vi "Resistor CalculatorLV2012 NIVerified.vi"() -> ()   [LabVIEW 2012]
doc: "This VI will calculate the value of your resistor based on the colors of the bands on your resistor. Each tab will show the meaning of each band of your resistor. When you are finished, you will find the nominal value of the resistor, the tolerance value on your resistor, the change in resistance caused by temperature and the maximum and minimum values that your resistance can be. \n\n1.) Select your resistor style from the tabs above.\n2.) Select the specific colors that are on your resistor.\n3.) If you are using a 6 Band resistor, enter the operating temperature of the resistor to determine the additional resistance caused by the change in temperature.\n4.) Click \"Calculate\" to determine the resulting resistor values."
panel:
  in  "Stop":bool
  in  "Calculate":bool
  in  "Tab Control":T1(tab)
  in  "1st Digit":u16(ring)=1 items=["Black", "Brown", "Red", "Orange", "Yellow", "Green", "Blue", "Purple", "Grey", "White"]
  in  "2nd Digit":u16(ring)=1 items=["Black", "Brown", "Red", "Orange", "Yellow", "Green", "Blue", "Purple", "Grey", "White"]
  in  "Multiplier":dbl(ring)=10.0 items=["Silver"=0.01, "Gold"=0.1, "Black"=1.0, "Brown"=10.0, "Red"=100.0, "Orange"=1000.0, "Yellow"=10000.0, "Green"=100000.0, "Blue"=1000000.0, "Purple"=10000000.0]
  in  "Tolerance":dbl(ring)=0.01 items=["Silver"=0.1, "Gold"=0.05, "Brown"=0.01, "Red"=0.02, "Green"=0.005, "Blue"=0.0025, "Purple"=0.001]
  out "1":bool
  out "2":bool
  out "Mult":bool
  out "Tol":bool
  out "Mult 2":bool
  out "1 2":bool
  out "2 2":bool
  out "3 2":bool
  out "Tol 2":bool
  in  "1st Digit":u16(ring)=1 items=["Black", "Brown", "Red", "Orange", "Yellow", "Green", "Blue", "Purple", "Grey", "White"]
  in  "2nd Digit":u16(ring)=1 items=["Black", "Brown", "Red", "Orange", "Yellow", "Green", "Blue", "Purple", "Grey", "White"]
  in  "Multiplier":dbl(ring)=10.0 items=["Silver"=0.01, "Gold"=0.1, "Black"=1.0, "Brown"=10.0, "Red"=100.0, "Orange"=1000.0, "Yellow"=10000.0, "Green"=100000.0, "Blue"=1000000.0, "Purple"=10000000.0]
  in  "Tolerance":dbl(ring)=0.01 items=["Silver"=0.1, "Gold"=0.05, "Brown"=0.01, "Red"=0.02, "Green"=0.005, "Blue"=0.0025, "Purple"=0.001]
  in  "3rd Digit":u16(ring)=1 items=["Black", "Brown", "Red", "Orange", "Yellow", "Green", "Blue", "Purple", "Grey", "White"]
  in  "Temperature (C)":dbl=25.0
  out "Temp 3":bool
  out "Mult 3":bool
  out "1 3":bool
  out "23":bool
  out "33":bool
  out "Tol 3":bool
  in  "1st Digit":u16(ring)=1 items=["Black", "Brown", "Red", "Orange", "Yellow", "Green", "Blue", "Purple", "Grey", "White"]
  in  "2nd Digit":u16(ring)=1 items=["Black", "Brown", "Red", "Orange", "Yellow", "Green", "Blue", "Purple", "Grey", "White"]
  in  "Multiplier":dbl(ring)=10.0 items=["Silver"=0.01, "Gold"=0.1, "Black"=1.0, "Brown"=10.0, "Red"=100.0, "Orange"=1000.0, "Yellow"=10000.0, "Green"=100000.0, "Blue"=1000000.0, "Purple"=10000000.0]
  in  "Tolerance":dbl(ring)=0.01 items=["Silver"=0.1, "Gold"=0.05, "Brown"=0.01, "Red"=0.02, "Green"=0.005, "Blue"=0.0025, "Purple"=0.001]
  in  "3rd Digit":u16(ring)=1 items=["Black", "Brown", "Red", "Orange", "Yellow", "Green", "Blue", "Purple", "Grey", "White"]
  in  "Temp Coefficient":i32(ring)=100 items=["Brown"=100, "Red"=50, "Orange"=15, "Yellow"=25, "Blue"=10, "Purple"=5]
  out "Resistor Value":dbl=110.0 format="%#_6p"
  out "Tolerance Value":dbl=1.1 format="%#_6p"
  out "Lowest Actual Value":dbl=108.9 format="%#_6p"
  out "Highest Actual Value":dbl=111.1 format="%#_6p"
  out "Temp Adjustment":dbl format="%#_6p"
  # "Overview: To demonstrate how to set up a simple analog window\nRequirement: LabVIEW Full Development System\nSteps:\n1. Choose how many bands do you want to calculate\n2. Set the color.\n3. Run the VI"
  # "This VI will calculate the value of your resistor based on the colors of the bands on your resistor. Each tab will show the meaning of each band of your resistor. When you are finished, you will find the nominal value of the resistor, the tolerance value on your resistor, the change in resistance caused by temperature and the maximum and minimum values that your resistance can be. \n\n1.) Select your resistor style from the tabs above.\n2.) Select the specific colors that are on your resistor.\n3.) If you are using a 6 Band resistor, enter the operating temperature of the resistor to determine the additional resistance caused by the change in temperature.\n4.) Click \"Calculate\" to determine the resulting resistor values."
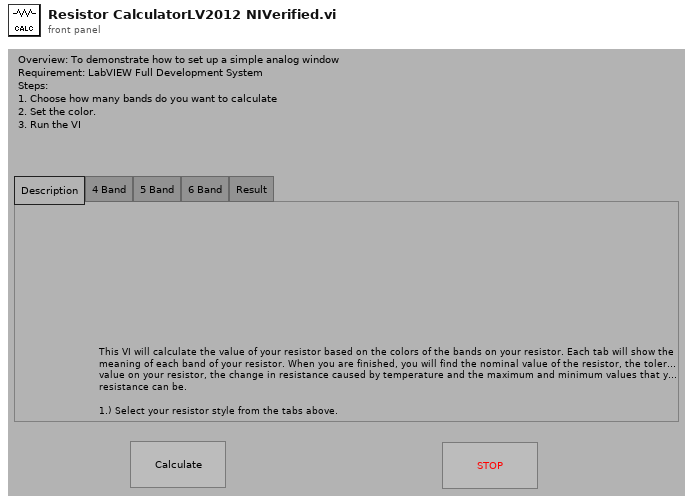
[diagram p1: front panel]
types:
  T1 = enum32{"Description", "4 Band", "5 Band", "6 Band", "Result"}
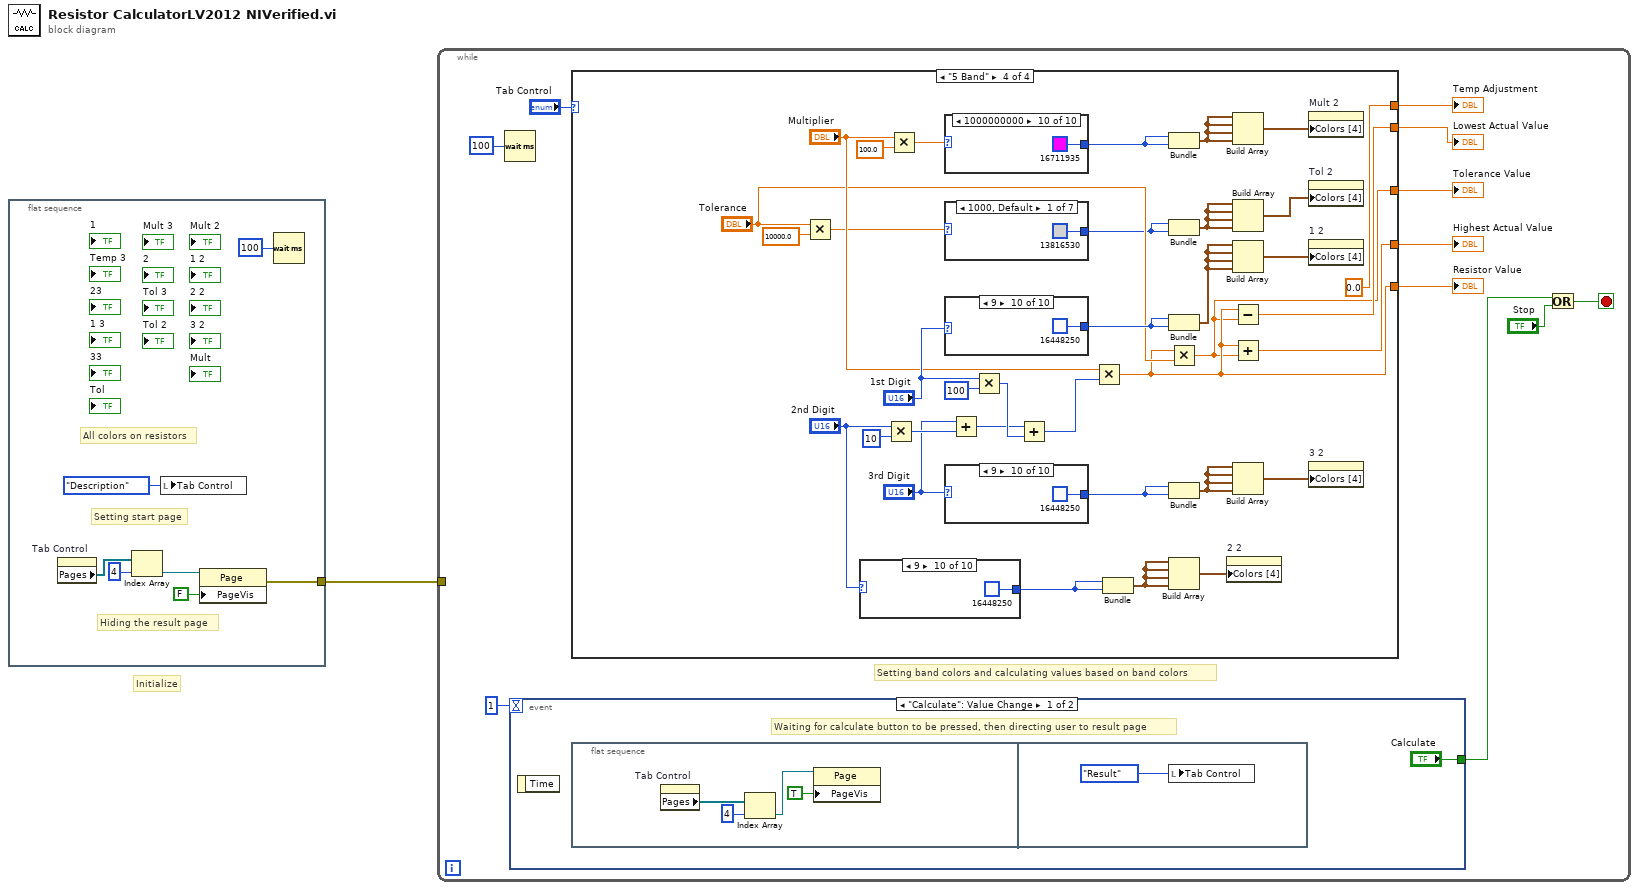
[diagram p0: block diagram]
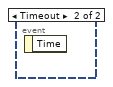
[diagram p2: hidden frame]
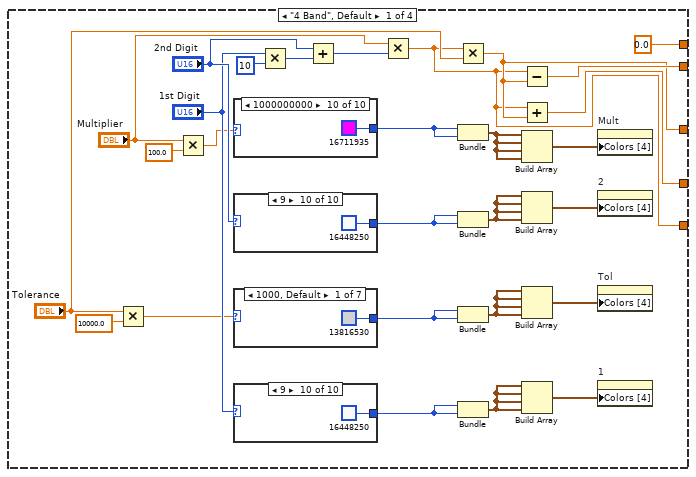
[diagram p3: hidden frame]
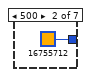
[diagram p4: hidden frame]
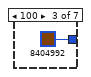
[diagram p5: hidden frame]
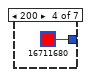
[diagram p6: hidden frame]
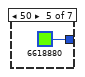
[diagram p7: hidden frame]
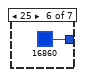
[diagram p8: hidden frame]
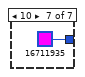
[diagram p9: hidden frame]
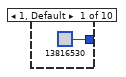
[diagram p10: hidden frame]
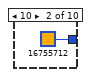
[diagram p11: hidden frame]
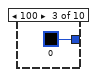
[diagram p12: hidden frame]
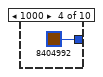
[diagram p13: hidden frame]
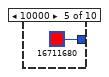
[diagram p14: hidden frame]
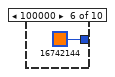
[diagram p15: hidden frame]
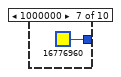
[diagram p16: hidden frame]
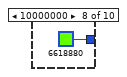
[diagram p17: hidden frame]
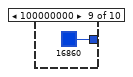
[diagram p18: hidden frame]
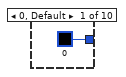
[diagram p19: hidden frame]
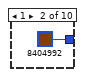
[diagram p20: hidden frame]
diagram:
  # "Initialize"
  n1 = flat-sequence {
    tunnel: [w2] -> w1
    frame #0 {
      # "Hiding the result page"
      # "Setting start page"
      # "All colors on resistors"
      n2 = property on="Tab Control" class="TabCtl (strict)"() -> ("Pages"=w3:refnum<vi>[])  [unwired: 2 in, 2 out]
      n3 = Index Array(array=w3, index=4) -> (element=w4:refnum<vi>)
      n4 = local write "Tab Control"(T1."Description" ("Tab Control")) -> ()
      n5 = property class="Page"(reference=w4, "PageVis"=FALSE ("Page Visible")) -> (error out=w2:errorcluster)  [unwired: 1 in, 1 out]
      n6 = Wait (ms)(milliseconds to wait=u32 100) -> ()  [unwired: 1 out]
    }
  }
  n7 = while {
    tunnel: w1 -> [_]
    stop <- w10 stop-if-true
    # "Setting band colors and calculating values based on band colors"
    n8 = Wait (ms)(milliseconds to wait=u32 100) -> ()  [unwired: 1 out]
    n9 = event shown="[0] \"Calculate\": Value Change" {
      selector: _ -> [_ _]
      dyn-events: _ -> [_ _]
      timeout: 1 -> [_ _]
      tunnel: ["Calculate" _] -> w18
      event "Calculate": Value Change {
        # "Waiting for calculate button to be pressed, then directing user to result page"
        n10 = event-data() -> ()  [unwired: 1 in, 1 out]
        n11 = flat-sequence {
          frame #0 {
            n12 = property on="Tab Control" class="TabCtl (strict)"() -> ("Pages"=w24:refnum<vi>[])  [unwired: 2 in, 2 out]
            n13 = Index Array(array=w24, index=4) -> (element=w23:refnum<vi>)
            n14 = property class="Page"(reference=w23, "PageVis"=TRUE ("Page Visible")) -> ()  [unwired: 1 in, 2 out]
          }
          frame #1 {
            n15 = local write "Tab Control"(T1."Result" ("Tab Control")) -> ()
          }
        }
      }
      event Timeout {
        n16 = event-data() -> ()  [unwired: 1 in, 1 out]
      }
    }
    n17 = case shown="\"5 Band\"" "Tab Control" {
      tunnel: [w30 w107 w186 w200] -> w17
      tunnel: [w29 w106 w186 w199] -> w16
      tunnel: [w28 w105 w186 w198] -> w15
      tunnel: [w27 w98 w186 w201] -> w14
      tunnel: [0.0 w100 w186 0.0] -> w13
      frame "4 Band", Default {
        n18 = Multiply(x="Tolerance", y=10000.0) -> (x*y=w36:dbl)
        n19 = Multiply(x="Multiplier", y=100.0) -> (x*y=w37:dbl)
        n20 = case shown="1000000000" w37 {
          tunnel: [u32 13816530 ("Color Box") u32 16755712 ("Color Box") u32 0 ("Color Box") u32 8404992 ("Color Box") u32 16711680 ("Color Box") u32 16742144 ("Color Box") u32 16776960 ("Color Box") u32 6618880 ("Color Box") u32 16860 ("Color Box") u32 16711935 ("Color Box")] -> w40
          frame 1, Default {
          }
          frame 10 {
          }
          frame 100 {
          }
          frame 1000 {
          }
          frame 10000 {
          }
          frame 100000 {
          }
          frame 1000000 {
          }
          frame 10000000 {
          }
          frame 100000000 {
          }
          frame 1000000000 {
          }
        }
        n21 = case shown="9" "2nd Digit" {
          tunnel: [u32 0 ("Color Box") u32 8404992 ("Color Box") u32 16711680 ("Color Box") u32 16742144 ("Color Box") u32 16776960 ("Color Box") u32 6618880 ("Color Box") u32 16860 ("Color Box") u32 16711935 ("Color Box") u32 12369084 ("Color Box") u32 16448250 ("Color Box")] -> w46
          frame 0, Default {
          }
          frame 1 {
          }
          frame 2 {
          }
          frame 3 {
          }
          frame 4 {
          }
          frame 5 {
          }
          frame 6 {
          }
          frame 7 {
          }
          frame 8 {
          }
          frame 9 {
          }
        }
        n22 = case shown="1000, Default" w36 {
          tunnel: [u32 13816530 ("Color Box") u32 16755712 ("Color Box") u32 8404992 ("Color Box") u32 16711680 ("Color Box") u32 6618880 ("Color Box") u32 16860 ("Color Box") u32 16711935 ("Color Box")] -> w32
          frame 1000, Default {
          }
          frame 500 {
          }
          frame 100 {
          }
          frame 200 {
          }
          frame 50 {
          }
          frame 25 {
          }
          frame 10 {
          }
        }
        n23 = case shown="9" "1st Digit" {
          tunnel: [u32 0 ("Color Box") u32 8404992 ("Color Box") u32 16711680 ("Color Box") u32 16742144 ("Color Box") u32 16776960 ("Color Box") u32 6618880 ("Color Box") u32 16860 ("Color Box") u32 16711935 ("Color Box") u32 12369084 ("Color Box") u32 16448250 ("Color Box")] -> w50
          frame 0, Default {
          }
          frame 1 {
          }
          frame 2 {
          }
          frame 3 {
          }
          frame 4 {
          }
          frame 5 {
          }
          frame 6 {
          }
          frame 7 {
          }
          frame 8 {
          }
          frame 9 {
          }
        }
        n24 = Multiply(x="1st Digit", y=10) -> (x*y=w52:i32)
        n25 = Add(x="2nd Digit", y=w52) -> (x+y=w51:i32)
        n26 = Multiply(x="Multiplier", y=w51) -> (x*y=w27:dbl)
        n27 = Multiply(x=w27, y="Tolerance") -> (x*y=w28:dbl)
        n28 = Bundle("Color Box"=w40, "Color Box"=w40) -> (w39:cluster{"Color Box":u32, "Color Box":u32})  [unwired: 1 in]
        n29 = Bundle("Color Box"=w46, "Color Box"=w46) -> (w47:cluster{"Color Box":u32, "Color Box":u32})  [unwired: 1 in]
        n30 = Bundle("Color Box"=w32, "Color Box"=w32) -> (w33:cluster{"Color Box":u32, "Color Box":u32})  [unwired: 1 in]
        n31 = Bundle("Color Box"=w50, "Color Box"=w50) -> (w49:cluster{"Color Box":u32, "Color Box":u32})  [unwired: 1 in]
        n32 = Subtract(x=w27, y=w28) -> (x-y=w29:dbl)
        n33 = Add(x=w27, y=w28) -> (x+y=w30:dbl)
        n34 = Build Array(w39, w39, w39, w39) -> (w38:cluster{"Color Box":u32, "Color Box":u32}[])
        n35 = Build Array(w47, w47, w47, w47) -> (w45:cluster{"Color Box":u32, "Color Box":u32}[])
        n36 = Build Array(w33, w33, w33, w33) -> (w31:cluster{"Color Box":u32, "Color Box":u32}[])
        n37 = Build Array(w49, w49, w49, w49) -> (w48:cluster{"Color Box":u32, "Color Box":u32}[])
        n38 = property on="Mult" class="Bool (strict)"("Colors [4]"=w38) -> ()  [unwired: 2 in, 2 out]
        n39 = property on="2" class="Bool (strict)"("Colors [4]"=w45) -> ()  [unwired: 2 in, 2 out]
        n40 = property on="Tol" class="Bool (strict)"("Colors [4]"=w31) -> ()  [unwired: 2 in, 2 out]
        n41 = property on="1" class="Bool (strict)"("Colors [4]"=w48) -> ()  [unwired: 2 in, 2 out]
      }
      frame "6 Band" {
        n42 = case shown="9" "2nd Digit" {
          tunnel: [u32 0 ("Color Box") u32 8404992 ("Color Box") u32 16711680 ("Color Box") u32 16742144 ("Color Box") u32 16776960 ("Color Box") u32 6618880 ("Color Box") u32 16860 ("Color Box") u32 16711935 ("Color Box") u32 12369084 ("Color Box") u32 16448250 ("Color Box")] -> w127
          frame 0, Default {
          }
          frame 1 {
          }
          frame 2 {
          }
          frame 3 {
          }
          frame 4 {
          }
          frame 5 {
          }
          frame 6 {
          }
          frame 7 {
          }
          frame 8 {
          }
          frame 9 {
          }
        }
        n43 = Multiply(x="2nd Digit", y=10) -> (x*y=w93:i32)
        n44 = case shown="9" "3rd Digit" {
          tunnel: [u32 0 ("Color Box") u32 8404992 ("Color Box") u32 16711680 ("Color Box") u32 16742144 ("Color Box") u32 16776960 ("Color Box") u32 6618880 ("Color Box") u32 16860 ("Color Box") u32 16711935 ("Color Box") u32 12369084 ("Color Box") u32 16448250 ("Color Box")] -> w112
          frame 0, Default {
          }
          frame 1 {
          }
          frame 2 {
          }
          frame 3 {
          }
          frame 4 {
          }
          frame 5 {
          }
          frame 6 {
          }
          frame 7 {
          }
          frame 8 {
          }
          frame 9 {
          }
        }
        n45 = case shown="9" "1st Digit" {
          tunnel: [u32 0 ("Color Box") u32 8404992 ("Color Box") u32 16711680 ("Color Box") u32 16742144 ("Color Box") u32 16776960 ("Color Box") u32 6618880 ("Color Box") u32 16860 ("Color Box") u32 16711935 ("Color Box") u32 12369084 ("Color Box") u32 16448250 ("Color Box")] -> w131
          frame 0, Default {
          }
          frame 1 {
          }
          frame 2 {
          }
          frame 3 {
          }
          frame 4 {
          }
          frame 5 {
          }
          frame 6 {
          }
          frame 7 {
          }
          frame 8 {
          }
          frame 9 {
          }
        }
        n46 = Multiply(x="1st Digit", y=100) -> (x*y=w92:i32)
        n47 = Compound Arithmetic op=ADD("3rd Digit", w93, w92) -> (w91:i32)
        n48 = Multiply(x="Tolerance", y=10000.0) -> (x*y=w119:dbl)
        n49 = case shown="100, Default" "Temp Coefficient" {
          tunnel: [u32 8404992 ("Color Box") u32 16711680 ("Color Box") u32 16742144 ("Color Box") u32 16776960 ("Color Box") u32 16860 ("Color Box") u32 16711935 ("Color Box")] -> w103
          frame 100, Default {
          }
          frame 50 {
          }
          frame 15 {
          }
          frame 25 {
          }
          frame 10 {
          }
          frame 5 {
          }
        }
        n50 = Multiply(x="Multiplier", y=w91) -> (x*y=w98:dbl)
        n51 = Bundle("Color Box"=w127, "Color Box"=w127) -> (w128:cluster{"Color Box":u32, "Color Box":u32})  [unwired: 1 in]
        n52 = Multiply(x="Multiplier", y=100.0) -> (x*y=w120:dbl)
        n53 = Compound Arithmetic op=MULTIPLY("Temp Coefficient", "Temperature (C)", w98) -> (w95:dbl)
        n54 = case shown="1000000000" w120 {
          tunnel: [u32 13816530 ("Color Box") u32 16755712 ("Color Box") u32 0 ("Color Box") u32 8404992 ("Color Box") u32 16711680 ("Color Box") u32 16742144 ("Color Box") u32 16776960 ("Color Box") u32 6618880 ("Color Box") u32 16860 ("Color Box") u32 16711935 ("Color Box")] -> w122
          frame 1, Default {
          }
          frame 10 {
          }
          frame 100 {
          }
          frame 1000 {
          }
          frame 10000 {
          }
          frame 100000 {
          }
          frame 1000000 {
          }
          frame 10000000 {
          }
          frame 100000000 {
          }
          frame 1000000000 {
          }
        }
        n55 = case shown="1000, Default" w119 {
          tunnel: [u32 13816530 ("Color Box") u32 16755712 ("Color Box") u32 8404992 ("Color Box") u32 16711680 ("Color Box") u32 6618880 ("Color Box") u32 16860 ("Color Box") u32 16711935 ("Color Box")] -> w115
          frame 1000, Default {
          }
          frame 500 {
          }
          frame 100 {
          }
          frame 200 {
          }
          frame 50 {
          }
          frame 25 {
          }
          frame 10 {
          }
        }
        n56 = Build Array(w128, w128, w128, w128) -> (w126:cluster{"Color Box":u32, "Color Box":u32}[])
        n57 = Bundle("Color Box"=w112, "Color Box"=w112) -> (w113:cluster{"Color Box":u32, "Color Box":u32})  [unwired: 1 in]
        n58 = Bundle("Color Box"=w131, "Color Box"=w131) -> (w130:cluster{"Color Box":u32, "Color Box":u32})  [unwired: 1 in]
        n59 = property on="23" class="Bool (strict)"("Colors [4]"=w126) -> ()  [unwired: 2 in, 2 out]
        n60 = Build Array(w113, w113, w113, w113) -> (w114:cluster{"Color Box":u32, "Color Box":u32}[])
        n61 = Build Array(w130, w130, w130, w130) -> (w129:cluster{"Color Box":u32, "Color Box":u32}[])
        n62 = property on="33" class="Bool (strict)"("Colors [4]"=w114) -> ()  [unwired: 2 in, 2 out]
        n63 = property on="1 3" class="Bool (strict)"("Colors [4]"=w129) -> ()  [unwired: 2 in, 2 out]
        n64 = Divide(x=w95, y=1000000.0) -> (x/y=w100:dbl)
        n65 = Bundle("Color Box"=w103, "Color Box"=w103) -> (w104:cluster{"Color Box":u32, "Color Box":u32})  [unwired: 1 in]
        n66 = Add(x=w100, y=w98) -> (x+y=w99:dbl)
        n67 = Build Array(w104, w104, w104, w104) -> (w102:cluster{"Color Box":u32, "Color Box":u32}[])
        n68 = Bundle("Color Box"=w122, "Color Box"=w122) -> (w121:cluster{"Color Box":u32, "Color Box":u32})  [unwired: 1 in]
        n69 = Multiply(x=w98, y="Tolerance") -> (x*y=w105:dbl)
        n70 = Bundle("Color Box"=w115, "Color Box"=w115) -> (w116:cluster{"Color Box":u32, "Color Box":u32})  [unwired: 1 in]
        n71 = property on="Temp 3" class="Bool (strict)"("Colors [4]"=w102) -> ()  [unwired: 2 in, 2 out]
        n72 = Build Array(w121, w121, w121, w121) -> (w109:cluster{"Color Box":u32, "Color Box":u32}[])
        n73 = Subtract(x=w99, y=w105) -> (x-y=w106:dbl)
        n74 = Add(x=w99, y=w105) -> (x+y=w107:dbl)
        n75 = Build Array(w116, w116, w116, w116) -> (w108:cluster{"Color Box":u32, "Color Box":u32}[])
        n76 = property on="Mult 3" class="Bool (strict)"("Colors [4]"=w109) -> ()  [unwired: 2 in, 2 out]
        n77 = property on="Tol 3" class="Bool (strict)"("Colors [4]"=w108) -> ()  [unwired: 2 in, 2 out]
      }
      frame "Result" {
        w186 = 0.0
      }
      frame "5 Band" {
        n78 = Multiply(x="Tolerance", y=10000.0) -> (x*y=w206:dbl)
        n79 = case shown="9" "2nd Digit" {
          tunnel: [u32 0 ("Color Box") u32 8404992 ("Color Box") u32 16711680 ("Color Box") u32 16742144 ("Color Box") u32 16776960 ("Color Box") u32 6618880 ("Color Box") u32 16860 ("Color Box") u32 16711935 ("Color Box") u32 12369084 ("Color Box") u32 16448250 ("Color Box")] -> w214
          frame 0, Default {
          }
          frame 1 {
          }
          frame 2 {
          }
          frame 3 {
          }
          frame 4 {
          }
          frame 5 {
          }
          frame 6 {
          }
          frame 7 {
          }
          frame 8 {
          }
          frame 9 {
          }
        }
        n80 = Multiply(x="2nd Digit", y=10) -> (x*y=w194:i32)
        n81 = Multiply(x="Multiplier", y=100.0) -> (x*y=w207:dbl)
        n82 = case shown="1000000000" w207 {
          tunnel: [u32 13816530 ("Color Box") u32 16755712 ("Color Box") u32 0 ("Color Box") u32 8404992 ("Color Box") u32 16711680 ("Color Box") u32 16742144 ("Color Box") u32 16776960 ("Color Box") u32 6618880 ("Color Box") u32 16860 ("Color Box") u32 16711935 ("Color Box")] -> w209
          frame 1, Default {
          }
          frame 10 {
          }
          frame 100 {
          }
          frame 1000 {
          }
          frame 10000 {
          }
          frame 100000 {
          }
          frame 1000000 {
          }
          frame 10000000 {
          }
          frame 100000000 {
          }
          frame 1000000000 {
          }
        }
        n83 = case shown="1000, Default" w206 {
          tunnel: [u32 13816530 ("Color Box") u32 16755712 ("Color Box") u32 8404992 ("Color Box") u32 16711680 ("Color Box") u32 6618880 ("Color Box") u32 16860 ("Color Box") u32 16711935 ("Color Box")] -> w202
          frame 1000, Default {
          }
          frame 500 {
          }
          frame 100 {
          }
          frame 200 {
          }
          frame 50 {
          }
          frame 25 {
          }
          frame 10 {
          }
        }
        n84 = case shown="9" "1st Digit" {
          tunnel: [u32 0 ("Color Box") u32 8404992 ("Color Box") u32 16711680 ("Color Box") u32 16742144 ("Color Box") u32 16776960 ("Color Box") u32 6618880 ("Color Box") u32 16860 ("Color Box") u32 16711935 ("Color Box") u32 12369084 ("Color Box") u32 16448250 ("Color Box")] -> w218
          frame 0, Default {
          }
          frame 1 {
          }
          frame 2 {
          }
          frame 3 {
          }
          frame 4 {
          }
          frame 5 {
          }
          frame 6 {
          }
          frame 7 {
          }
          frame 8 {
          }
          frame 9 {
          }
        }
        n85 = case shown="9" "3rd Digit" {
          tunnel: [u32 0 ("Color Box") u32 8404992 ("Color Box") u32 16711680 ("Color Box") u32 16742144 ("Color Box") u32 16776960 ("Color Box") u32 6618880 ("Color Box") u32 16860 ("Color Box") u32 16711935 ("Color Box") u32 12369084 ("Color Box") u32 16448250 ("Color Box")] -> w195
          frame 0, Default {
          }
          frame 1 {
          }
          frame 2 {
          }
          frame 3 {
          }
          frame 4 {
          }
          frame 5 {
          }
          frame 6 {
          }
          frame 7 {
          }
          frame 8 {
          }
          frame 9 {
          }
        }
        n86 = Add(x="3rd Digit", y=w194) -> (x+y=w191:i32)
        n87 = Multiply(x="1st Digit", y=100) -> (x*y=w220:i32)
        n88 = Add(x=w191, y=w220) -> (x+y=w219:i32)
        n89 = Multiply(x="Multiplier", y=w219) -> (x*y=w201:dbl)
        n90 = Bundle("Color Box"=w214, "Color Box"=w214) -> (w215:cluster{"Color Box":u32, "Color Box":u32})  [unwired: 1 in]
        n91 = Bundle("Color Box"=w209, "Color Box"=w209) -> (w208:cluster{"Color Box":u32, "Color Box":u32})  [unwired: 1 in]
        n92 = Bundle("Color Box"=w202, "Color Box"=w202) -> (w203:cluster{"Color Box":u32, "Color Box":u32})  [unwired: 1 in]
        n93 = Bundle("Color Box"=w218, "Color Box"=w218) -> (w217:cluster{"Color Box":u32, "Color Box":u32})  [unwired: 1 in]
        n94 = Multiply(x=w201, y="Tolerance") -> (x*y=w198:dbl)
        n95 = Bundle("Color Box"=w195, "Color Box"=w195) -> (w196:cluster{"Color Box":u32, "Color Box":u32})  [unwired: 1 in]
        n96 = Build Array(w215, w215, w215, w215) -> (w213:cluster{"Color Box":u32, "Color Box":u32}[])
        n97 = property on="2 2" class="Bool (strict)"("Colors [4]"=w213) -> ()  [unwired: 2 in, 2 out]
        n98 = Build Array(w208, w208, w208, w208) -> (w189:cluster{"Color Box":u32, "Color Box":u32}[])
        n99 = Build Array(w203, w203, w203, w203) -> (w188:cluster{"Color Box":u32, "Color Box":u32}[])
        n100 = Build Array(w217, w217, w217, w217) -> (w216:cluster{"Color Box":u32, "Color Box":u32}[])
        n101 = Subtract(x=w201, y=w198) -> (x-y=w199:dbl)
        n102 = Add(x=w201, y=w198) -> (x+y=w200:dbl)
        n103 = Build Array(w196, w196, w196, w196) -> (w197:cluster{"Color Box":u32, "Color Box":u32}[])
        n104 = property on="Mult 2" class="Bool (strict)"("Colors [4]"=w189) -> ()  [unwired: 2 in, 2 out]
        n105 = property on="Tol 2" class="Bool (strict)"("Colors [4]"=w188) -> ()  [unwired: 2 in, 2 out]
        n106 = property on="1 2" class="Bool (strict)"("Colors [4]"=w216) -> ()  [unwired: 2 in, 2 out]
        n107 = property on="3 2" class="Bool (strict)"("Colors [4]"=w197) -> ()  [unwired: 2 in, 2 out]
      }
    }
    "Highest Actual Value" <- w17
    "Lowest Actual Value" <- w16
    "Tolerance Value" <- w15
    "Resistor Value" <- w14
    "Temp Adjustment" <- w13
    n108 = Or(x=w18, y="Stop") -> (x .or. y?=w10:bool)
  }
